vi "Create Custom Errors.vi"(8 "error in":errorcluster, 11 "Custom Errors Info":T1[](array[typedef])) -> (0 "error out":errorcluster, 3 "Custom Errors out":refnum<class "Custom Errors.lvclass">)   [LabVIEW 2021, in "TAF Proj Document Type.lvlib" / "Custom Errors.lvclass"]
uses:
  <vilib>/Wovalab/AntiDoc/Document Type/Add-ons/LabVIEW TAF Project/Custom Errors/Custom Errors.lvclass
  C:/Program Files (x86)/National Instruments/LabVIEW 2021/vi.lib/Wovalab/AntiDoc/Bloc/Bloc.lvclass
  <vilib>/Wovalab/AntiDoc/Bloc/Raw Custom Error Info--cluster.ctl
  <vilib>/Wovalab/AntiDoc/Bloc/Custom Error Info--cluster.ctl
  <vilib>/Wovalab/AntiDoc/Bloc/Bloc.lvclass/Bloc.ctl
  <vilib>/Wovalab/AntiDoc/Document Type/Add-ons/LabVIEW TAF Project/Custom Errors/Custom Errors.lvclass/Custom Errors.ctl
  <vilib>/Wovalab/AntiDoc/Bloc/Write Name.vi
  <vilib>/Wovalab/AntiDoc/Bloc/Bloc.lvclass
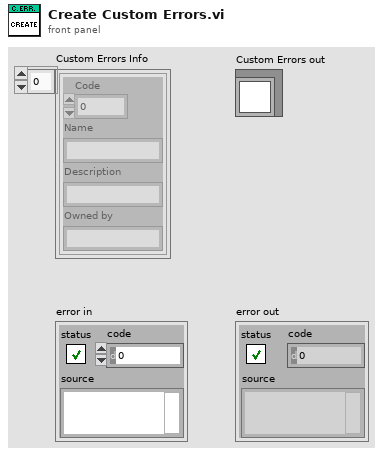
[diagram p1: front panel]
types:
  T1 = typedef "AntiDoc.lvlib/Bloc.lvclass/Raw Custom Error Info--cluster.ctl" = cluster{"Code":i32, "Name":string, "Description":string, "Owned by":string}
  T2 = typedef "AntiDoc.lvlib/Bloc.lvclass/Custom Error Info--cluster.ctl" = cluster{"Code":i32, "Name":string, "Description":string, "Owned By":string[]}
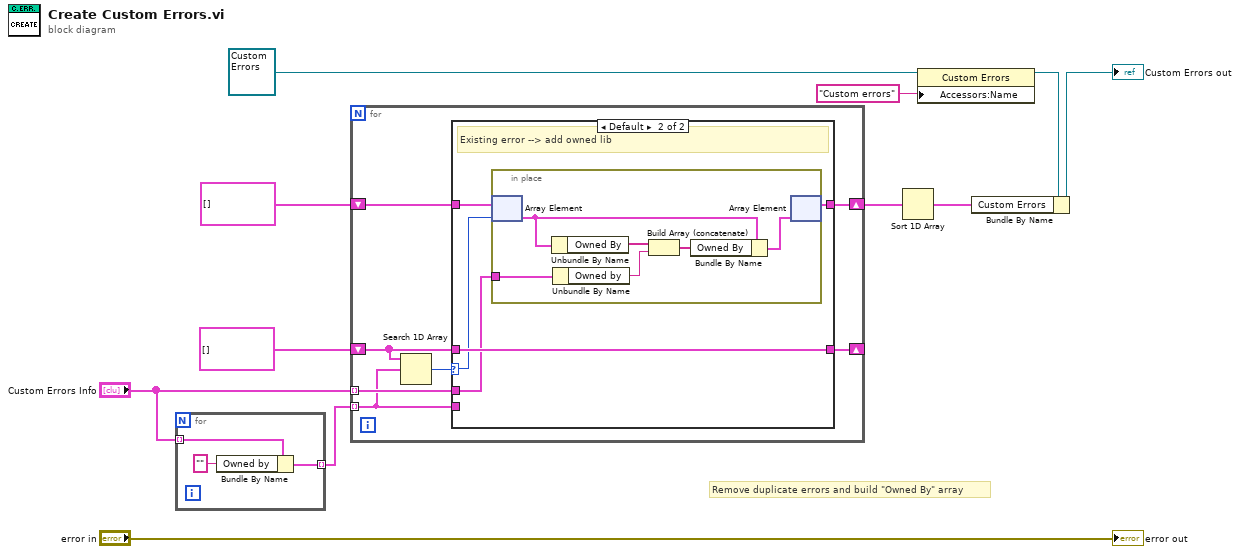
[diagram p0: block diagram]
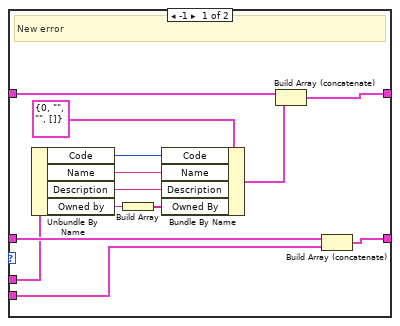
[diagram p2: hidden frame]
diagram:
  # "Remove duplicate errors and build \"Owned By\" array"
  n1 = for {
    tunnel: "Custom Errors Info" -> [w14] mode=indexing
    tunnel: [w12] -> w5 mode=indexing
    n2 = Bundle By Name(cluster=w14, "Owned by"="") -> (w12:T1)
  }
  n3 = for {
    tunnel: "Custom Errors Info" -> [w18] mode=indexing
    shift-right: [w19] -> w8
    shift-left: T2[] [] -> [w20]
    tunnel: w5 -> [w15] mode=indexing
    shift-right: [w16] -> _
    shift-left: T1[] [] ("Custom Errors Info") -> [w17]
    n4 = Search 1D Array(1D array=w17, element=w15) -> (index of element=w21:i32)  [unwired: 1 in]
    n5 = case shown="Default" w21 {
      selector: w21 -> [_ w36]
      tunnel: w20 -> [w34 w38]
      tunnel: w18 -> [w29 w35]
      tunnel: [w33 w37] -> w19
      tunnel: w17 -> [w32 w39]
      tunnel: [w31 w39] -> w16
      tunnel: w15 -> [w22 _]
      frame -1 {
        # "New error"
        n6 = Unbundle By Name(w29) -> ("Code"=w28:i32, "Name"=w27:string, "Description"=w26:string, "Owned by"=w25:string)
        n7 = Build Array(w25) -> (w24:string[])
        n8 = Bundle By Name(cluster=T2 {"Code"=0, "Name"="", "Description"="", "Owned By"=[]} ("Custom Error Info"), "Code"=w28, "Name"=w27, "Description"=w26, "Owned By"=w24) -> (w23:T2)
        n9 = Build Array (concatenate)(w34, w23) -> (w33:T2[])
        n10 = Build Array (concatenate)(w32, w22) -> (w31:T1[])
      }
      frame Default {
        # "Existing error --> add owned lib"
        n11 = in-place {
          in-place-border: w35 -> [w42]
          n12 = in-place-array #1(w38, w36) -> (w40:T2)
          n13 = Unbundle By Name(w40) -> ("Owned By"=w41:string[])
          n14 = Unbundle By Name(w42) -> ("Owned by"=w45:string)
          n15 = Build Array (concatenate)(w41, w45) -> (w44:string[])
          n16 = Bundle By Name(cluster=w40, "Owned By"=w44) -> (w43:T2)
          n17 = in-place-array #1(w43) -> (w37:T2[])  [unwired: 1 out]
        }
      }
    }
  }
  n18 = Sort 1D Array(array=w8) -> (sorted array=w7:T2[])
  n19 = property class="Custom Errors"(reference=refnum<class "Custom Errors.lvclass"> refnum ("Custom Errors in"), "Accessors:Name"="Custom errors" ("Title")) -> (reference out=w2:refnum<class "Custom Errors.lvclass">)  [unwired: 1 in, 1 out]
  n20 = Bundle By Name(cluster=w2, "Custom Errors"=w7) -> (→"Custom Errors out":refnum<class "Custom Errors.lvclass">)
  "error out" <- "error in"
